vi "CheckForEOL.vi"(11 "String":string) -> (3 "NOT EOL?":bool)   [LabVIEW 2017]
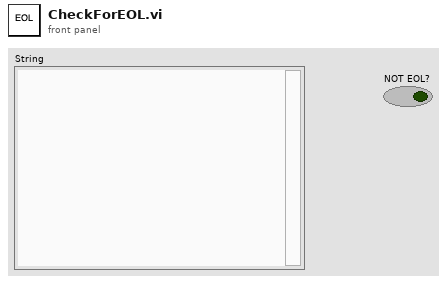
[diagram p1: front panel]
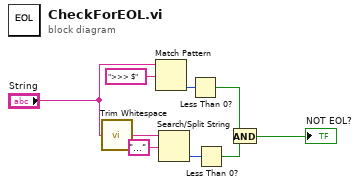
[diagram p0: block diagram]
diagram:
  n1 = call <vilib>:"Trim Whitespace.vi"("string"="String") -> ("trimmed string"=w9:string)  [unwired: 1 in]
  n2 = Match Pattern(string="String", regular expression=">>> $") -> (offset past match=w5:i32)  [unwired: 1 in, 3 out]
  n3 = Search/Split String(string=w9, search string/char (-)="..." ("regular expression")) -> (offset of match=w8:i32)  [unwired: 1 in, 2 out]
  n4 = Less Than 0?(x=w5) -> (x < 0?=w6:bool)
  n5 = Less Than 0?(x=w8) -> (x < 0?=w7:bool)
  n6 = And(x=w6, y=w7) -> (x .and. y?=→"NOT EOL?":bool)
